vi "Parse Parameter - URL.vi"(8 "error in (no error)":errorcluster, 11 "URL":string) -> (0 "error out":errorcluster, 3 "URL Parameters":T1[](array[typedef]))   [LabVIEW 2011, in "i3-oauth.lvlib"]
uses:
  i3-oauth.lvlib
  Controls/key-value-pairs.ctl
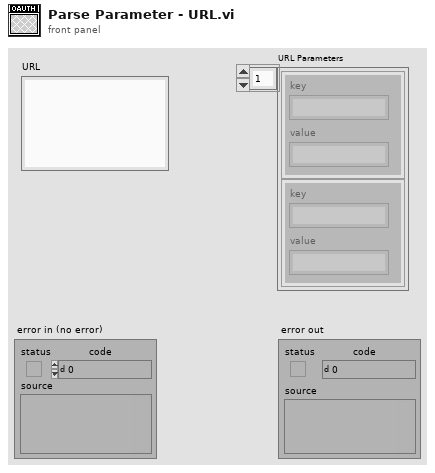
[diagram p1: front panel]
types:
  T1 = typedef "i3-oauth.lvlib/key-value-pairs.ctl" = cluster{"key":string, "value":string}
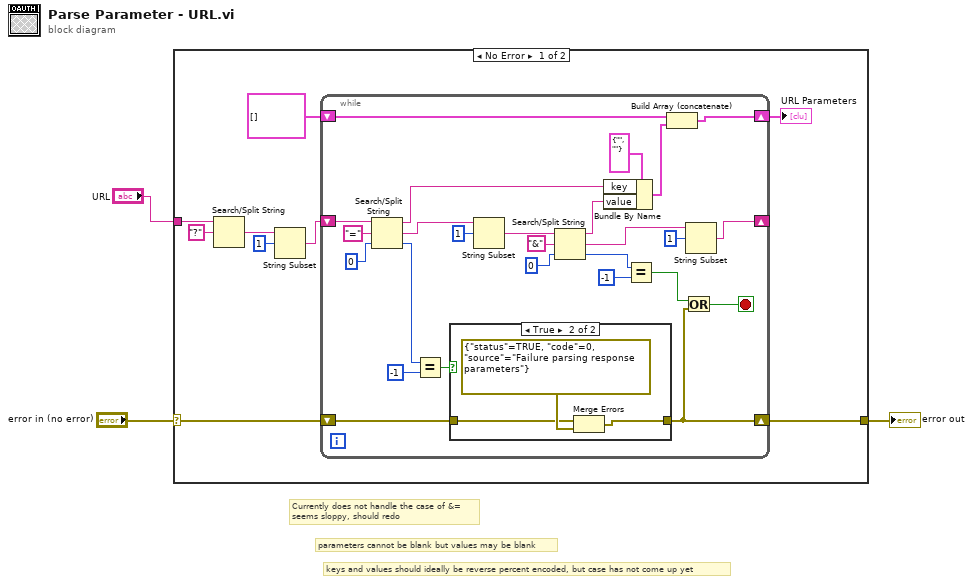
[diagram p0: block diagram]
diagram:
  # "keys and values should ideally be reverse percent encoded, but case has not come up yet"
  # "parameters cannot be blank but values may be blank"
  # "Currently does not handle the case of &=\nseems sloppy, should redo"
  n1 = case shown="No Error" "error in (no error)" {
    selector: "error in (no error)" -> [w10 w43]
    tunnel: "URL" -> [w8 _]
    tunnel: [w9 w43] -> w1
    frame No Error {
      n2 = Search/Split String(string=w8, search string/char (-)="?") -> (match + rest of string=w4:string)  [unwired: 1 in, 2 out]
      n3 = String Subset(string=w4, offset (0)=1) -> (substring=w5:string)  [unwired: 1 in]
      n4 = while {
        shift-right: [w30] -> w11
        shift-left: T1[] [] ("Body Parameters") -> [w32]
        shift-right: [w13] -> w9
        shift-left: w10 -> [w14]
        shift-right: [w17] -> _
        shift-left: w5 -> [w37]
        stop <- w25 stop-if-true
        n5 = Search/Split String(string=w37, search string/char (-)="=", offset (0)=0) -> (substring before match=w35:string, match + rest of string=w24:string, offset of match=w27:i32)
        n6 = Equal?(x=w27, y=-1) -> (x = y?=w15:bool)
        n7 = case shown="True" w15 {
          tunnel: w14 -> [w39 w41]
          tunnel: [w39 w40] -> w13
          frame False {
          }
          frame True {
            n8 = Merge Errors(w41, errorcluster {"status"=TRUE, "code"=0, "source"="Failure parsing response parameters"} ("error in (no error)")) -> (w40:errorcluster)
          }
        }
        n9 = String Subset(string=w24, offset (0)=1) -> (substring=w23:string)  [unwired: 1 in]
        n10 = Search/Split String(string=w23, search string/char (-)="&", offset (0)=0) -> (substring before match=w19:string, match + rest of string=w16:string, offset of match=w29:i32)
        n11 = Bundle By Name(cluster=T1 {"key"="", "value"=""} ("Key Value Pair"), "key"=w35, "value"=w19) -> (w31:T1)
        n12 = Equal?(x=w29, y=-1) -> (x = y?=w26:bool)
        n13 = Build Array (concatenate)(w32, w31) -> (w30:T1[])
        n14 = Or(x=w26, y=w13) -> (x .or. y?=w25:bool)
        n15 = String Subset(string=w16, offset (0)=1) -> (substring=w17:string)  [unwired: 1 in]
      }
      "URL Parameters" <- w11
    }
    frame Error {
    }
  }
  "error out" <- w1
